vi "CSGaussmeter.Reset.vi"(0 "i ref in":refnum<vi>, 11 "error in (no error)":errorcluster) -> (4 "i ref out":refnum<vi>, 15 "error out":errorcluster)   [LabVIEW 2014, in "CSGaussmeter.lvlib"]
doc: "The VI starts the function Reset. Max/Min or Peak sets to Zero.\n\n Durch die Funktion Reset wird MAX/MIN bzw. Peak auf Null gesetzt."
uses:
  CSGaussmeter.lvlib
  instr.lib/FH_55/TypeDef/Value_String.ctl
  CS_Core/CSObj/CSObj.lvlib
  CSlibraries/UtilityLib/UtilityLib.lvlib
  instr.lib/FH_55/FH 55.lvlib
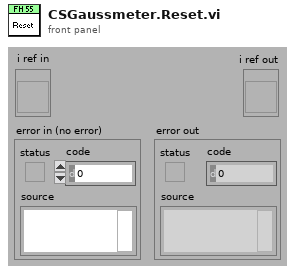
[diagram p1: front panel]
types:
  T1 = typedef "FH 55.lvlib/Value_String.ctl" = cluster{"Numeric":dbl, "String":string}
  T2 = typedef "CSGaussmeter.lvlib/CSGaussmeter.i attribute.ctl" = cluster{"Name":string, "VISA Resource Name":refnum<visa-resource-name>, "actValues":cluster{" Limit":bool, "Unit ":T3, "Temp_Unit":T4, "Max":T5, " Filter":bool, " Peak":bool, " Auto_Range":bool, "Range":T6, " Rel":bool, " CTemp":bool, " CField":bool, "AC_DC ":bool, "Set_lower":cluster{"Numeric":dbl, "Cancel Button":bool, "Unit":T7}, "Set_upper":cluster{"Numeric":dbl, "Cancel Button":bool, "Unit":T7}, "Set_Rel":cluster{"Numeric":dbl, "Cancel Button":bool, "Unit":T7}, "Zero":bool, " Local":bool, "Reset":bool, " Init":bool}, "FH 55 Gauss-/Teslameter":T8, "MAX_Value":T1, "MIN_Value":T1, "Rel_Value":T1, "Array ":string[], "LIMU":dbl, " LIML":dbl, "Messwerte 2":string, "Messwerte ":cluster{"Numeric":i32, "OK Button":bool}, "serviceID":cluster{"Current ID":i32, "Unit ID":i32, "Temp ID":i32, "Name ID \n":i32, "Visa ID ":i32}, "setValues ":cluster{" Limit":bool, "Unit ":T3, "Temp_Unit":T4, "Max":T5, " Filter":bool, " Peak":bool, " Auto_Range":bool, "Range":T6, " Rel":bool, " CTemp":bool, " CField":bool, "AC_DC ":bool, "Set_lower":cluster{"Numeric":dbl, "Cancel Button":bool, "Unit":T7}, "Set_upper":cluster{"Numeric":dbl, "Cancel Button":bool, "Unit":T7}, "Set_Rel":cluster{"Numeric":dbl, "Cancel Button":bool, "Unit":T7}, "Zero":bool, " Local":bool, "Reset":bool, " Init":bool}}
  T3 = typedef "FH 55.lvlib/Unit.ctl" = enum16{"T", "G", "A/m"}
  T4 = typedef "FH 55.lvlib/Temp_Unit.ctl" = enum16{"Temp off", "Celsius", "Fahrenheit"}
  T5 = typedef "FH 55.lvlib/Max.ctl" = enum16{"MAX off", "Show MAX", "MAX/MIN"}
  T6 = typedef "FH 55.lvlib/Range.ctl" = enum16{"1", "2", "3", "4", "5", "6", "7"}
  T7 = typedef "FH 55.lvlib/Unit2.ctl" = enum16{"mT", "G", "kA/m"}
  T8 = typedef "FH 55.lvlib/Display.ctl" = cluster{"current value":string, "Limit":string, "Remote":string, "function ":string, "Cluster":cluster{"AC/DC":string, "Auto":string, "Filter":string, "Range":string, "Rel":string, "Peak":string}}
  T9 = cluster{"VISA Resource Name":refnum<visa-resource-name>}
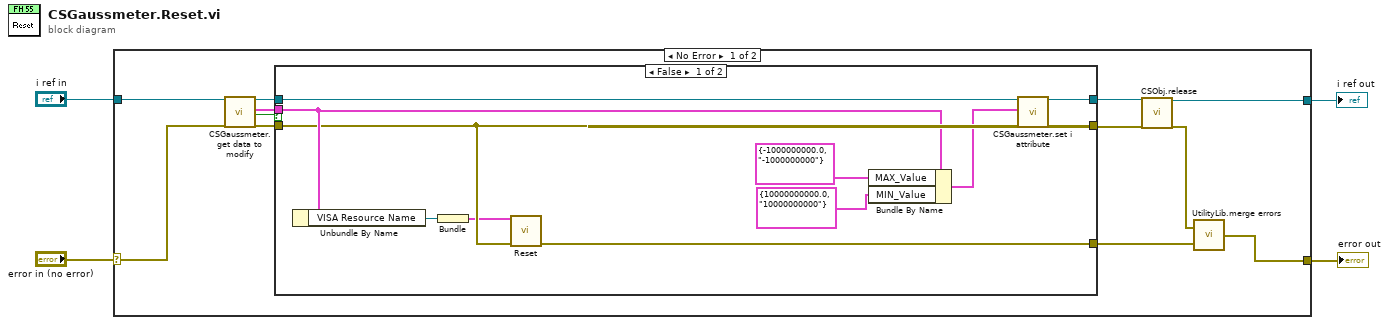
[diagram p0: block diagram]
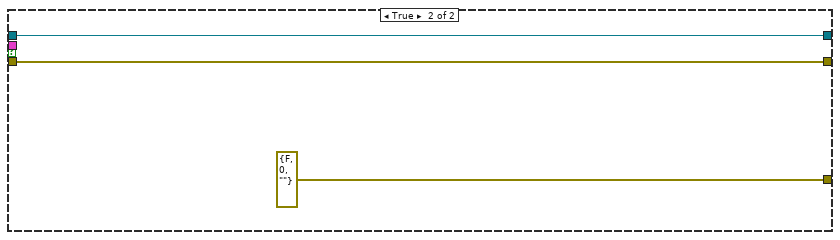
[diagram p2: hidden frame]
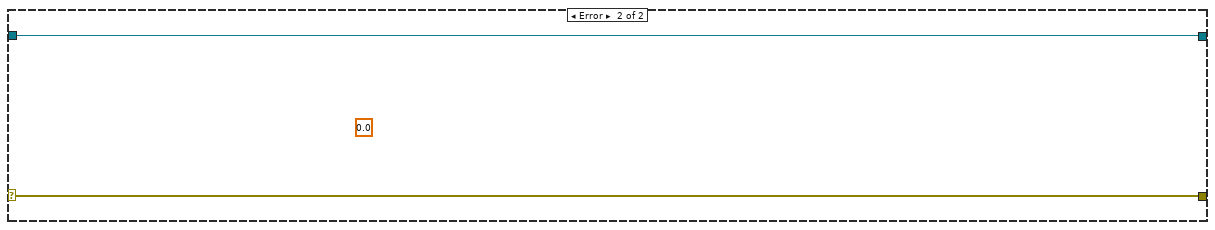
[diagram p3: hidden frame]
diagram:
  n1 = case shown="No Error" "error in (no error)" {
    selector: "error in (no error)" -> [w11 w30]
    tunnel: [w12 w30] -> w1
    tunnel: "i ref in" -> [w10 w31]
    tunnel: [w5 w31] -> w2
    frame No Error {
      n2 = call "CSGaussmeter.get data to modify.vi"("i ref in"=w10, "error in (no error)"=w11) -> ("i ref out"=w9:refnum<vi>, "i attribute"=w8:T2, "timed out"=w7:bool, "error out"=w6:errorcluster)  [unwired: 14 in]
      n3 = case shown="False" w7 {
        tunnel: w9 -> [w24 w28]
        tunnel: w6 -> [w21 w29]
        tunnel: w8 -> [w25 _]
        tunnel: [w21 w29] -> w14
        tunnel: [w22 w28] -> w16
        tunnel: [w19 errorcluster {"status"=FALSE, "code"=0, "source"=""} ("error out")] -> w13
        frame False {
          n4 = Unbundle By Name(w25) -> ("VISA Resource Name"=w26:refnum<visa-resource-name>)
          n5 = Bundle("VISA Resource Name"=w26) -> (w20:T9)  [unwired: 1 in]
          n6 = call "Reset.vi"("VisaCluster"=w20, "error in (no error)"=w21) -> ("error out"=w19:errorcluster)  [unwired: 11 in, 2 out]
          n7 = Bundle By Name(cluster=w25, "MAX_Value"=T1 {"Numeric"=-1000000000.0, "String"="-1000000000"}, "MIN_Value"=T1 {"Numeric"=10000000000.0, "String"="10000000000"}) -> (w23:T2)
          n8 = call "CSGaussmeter.set i attribute.vi"("i ref in"=w24, "i attribute"=w23) -> ("i ref out"=w22:refnum<vi>)  [unwired: 16 in, 1 out]
        }
        frame True {
        }
      }
      n9 = call "CSObj.release.vi"("i ref in"=w16, "error in (no error)"=w14) -> ("i ref out"=w5:refnum<vi>, "error out"=w15:errorcluster)  [unwired: 16 in]
      n10 = call "UtilityLib.merge errors.vi"("error2 (no error)"=w13, "error1 (no error)"=w15) -> ("error out"=w12:errorcluster)
    }
    frame Error {
      (unwired) 0.0 ("Mid Setting [A or T]")
    }
  }
  "i ref out" <- w2
  "error out" <- w1
